vi "setRange.vi"(0 "Interface in":T2, 5 "Ranges":T1, 11 "error in":errorcluster) -> (4 "Interface out":T2, 15 "error out":errorcluster)   [LabVIEW 2017, in "AFE_interface.lvlib"]
uses:
  AFE_interface.lvlib
  InterfaceRef.ctl
  <instrlib>/_niInstr/Instruction Framework/v1/Host/Instruction Target/niInstr Instruction Target v1 Host.lvclass
  <instrlib>/_niInstr/Instruction Framework/v1/Host/Instruction Framework Context/niInstr Instruction Framework Context v1 Host.lvclass
  AFE/Range.ctl
  AFE/ActiveFrontEnd.lvlib
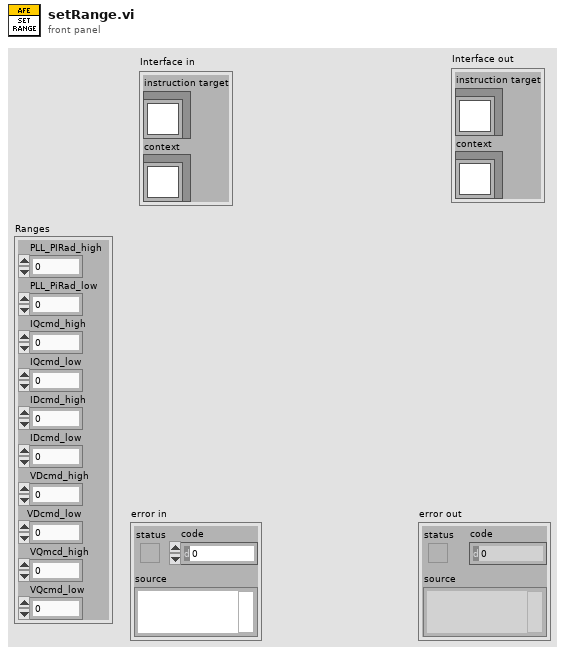
[diagram p1: front panel]
types:
  T1 = typedef "ActiveFrontEnd.lvlib/Range.ctl" = cluster{"PLL_PIRad_high":sgl, "PLL_PiRad_low":sgl, "IQcmd_high":sgl, "IQcmd_low":sgl, "IDcmd_high":sgl, "IDcmd_low":sgl, "VDcmd_high":sgl, "VDcmd_low":sgl, "VQmcd_high":sgl, "VQcmd_low":sgl}
  T2 = typedef "AFE_interface.lvlib/InterfaceRef.ctl" = cluster{"instruction target":refnum<class "niInstr Instruction Target v1 Host.lvclass">, "context":refnum<class "niInstr Instruction Framework Context v1 Host.lvclass">}
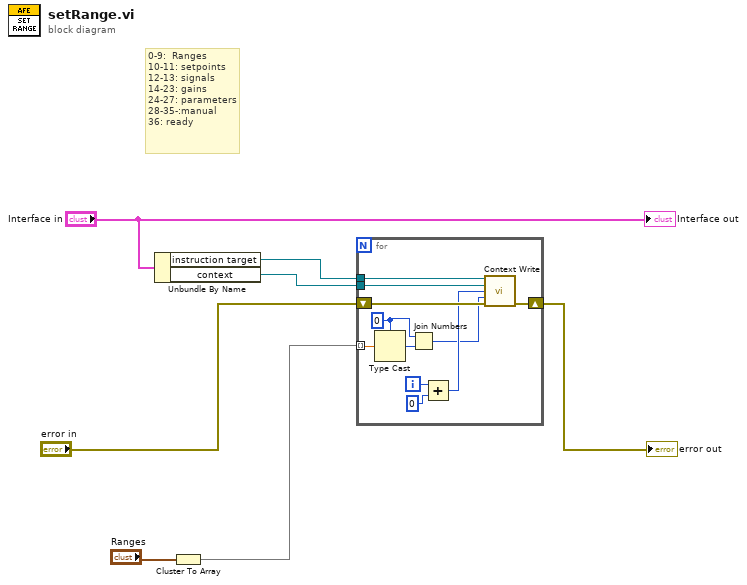
[diagram p0: block diagram]
diagram:
  # "0-9:  Ranges\n10-11: setpoints\n12-13: signals\n14-23: gains\n24-27: parameters\n28-35-:manual\n36: ready"
  n1 = Unbundle By Name("Interface in") -> ("instruction target"=w6:refnum<class "niInstr Instruction Target v1 Host.lvclass">, "context"=w5:refnum<class "niInstr Instruction Framework Context v1 Host.lvclass">)
  n2 = Cluster To Array(cluster="Ranges") -> (array=w1:sgl[])
  n3 = for {
    tunnel: w6 -> [w18]
    tunnel: w5 -> [w17]
    shift-right: [w15] -> w3
    shift-left: "error in" -> [w16]
    tunnel: w1 -> [w11] mode=indexing
    i -> [w12]
    w10 = u32 0
    n4 = Type Cast(type=w10, x=w11) -> (*(type *) &x=w9:u32)
    n5 = Join Numbers(hi=w10, lo=w9) -> ((hi.lo)=w8:u64)
    n6 = Add(x=w12, y=0) -> (x+y=w13:i32)
    n7 = call <instrlib>:"Context Write.vi"("instruction target in"=w18, "context in"=w17, "address"=w13, "data"=w8, "error in"=w16) -> ("error out"=w15:errorcluster)  [unwired: 8 in, 2 out]
  }
  "error out" <- w3
  "Interface out" <- "Interface in"
